vi "Create image name.vi"(8 "error in (no error)":errorcluster, 9 "Suffix":string, 10 "Channel":u8, 11 "Simulated_CCD_Camera in":refnum<class "Simulated_CCD_Camera.lvclass">) -> (0 "error out":errorcluster, 3 "Simulated_CCD_Camera out":refnum<class "Simulated_CCD_Camera.lvclass">)   [LabVIEW 2018, in "Simulated_CCD_Camera.lvclass"]
doc: "Create the image name\n\nThis name is composed by the following parts. First, there are the year, month, and day of the beginning of the night in the format YYYYMMDD. Second, there is the string s4cx, where x is the number of the channel. Then, there is the image index in the format 000000. This index is incremented after each acquisition. Finally, there is the suffix provided by the user. Following, there is an example of the image name\n\n20230101_s4c1_000001_zero.fits"
uses:
  Simulated_CCD_Camera.lvclass
  Simulated_CCD_Camera.lvclass/Simulated_CCD_Camera.ctl
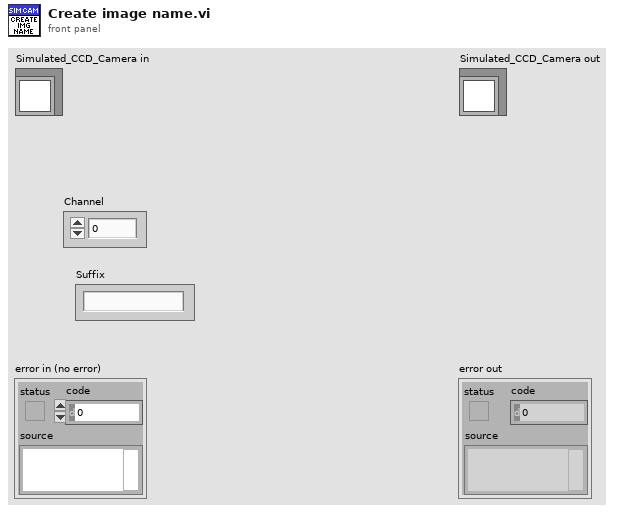
[diagram p1: front panel]
types:
  T1 = typedef "LVDateTimeRec.ctl" = cluster{"fractional second":dbl, "second":i32, "minute":i32, "hour":i32, "day of month":i32, "month":i32, "year":i32, "day of week":i32, "day of year":i32, "DST":i32}
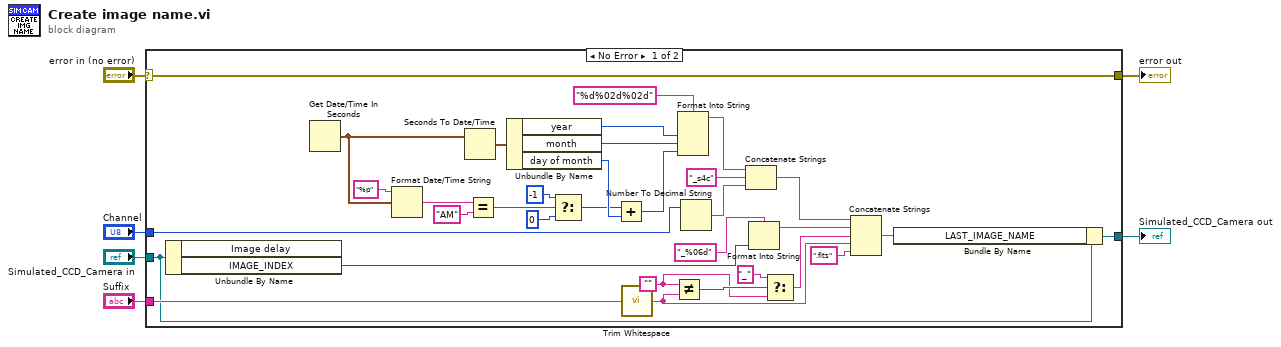
[diagram p0: block diagram]
diagram:
  n1 = case shown="No Error" "error in (no error)" {
    selector: "error in (no error)" -> [w11 w41]
    tunnel: [w11 w41] -> w5
    tunnel: [w29 w40] -> w3
    tunnel: "Simulated_CCD_Camera in" -> [w30 w40]
    tunnel: "Suffix" -> [w32 _]
    tunnel: "Channel" -> [w31 _]
    frame No Error {
      w26 = ""
      n2 = Unbundle By Name(w30) -> ("IMAGE_INDEX"=w22:u32)  [unwired: 1 out]
      n3 = Get Date/Time In Seconds() -> (seconds since 1Jan1904=w12:timestamp)
      n4 = Format Date/Time String(time format string (%c)="%p", seconds (now)=w12) -> (date/time string=w14:string)  [unwired: 1 in]
      n5 = Seconds To Date/Time(time stamp (now)=w12) -> (date time rec=w25:T1)  [unwired: 1 in]
      n6 = Equal?(x=w14, y="AM") -> (x = y?=w15:bool)
      n7 = Unbundle By Name(w25) -> ("year"=w24:i32, "month"=w23:i32, "day of month"=w19:i32)
      n8 = Select(t=-1, s=w15, f=0) -> (s? t:f=w18:i32)
      n9 = Add(x=w18, y=w19) -> (x+y=w17:i32)
      n10 = call <vilib>:"Trim Whitespace.vi"("string"=w32) -> ("trimmed string"=w9:string)  [unwired: 1 in]
      n11 = Not Equal?(x=w26, y=w9) -> (x != y?=w36:bool)
      n12 = Format Into String(format string="%d%02d%02d", w24, w23, w17) -> (resulting string=w27:string)  [unwired: 2 in, 1 out]
      n13 = Number To Decimal String(number=w31) -> (decimal integer string=w38:string)  [unwired: 1 in]
      n14 = Concatenate Strings(w27, "_s4c" ("string"), w38) -> (w37:string)
      n15 = Format Into String(format string="_%06d", w22) -> (resulting string=w8:string)  [unwired: 2 in, 1 out]
      n16 = Select(t="_" ("string"), s=w36, f=w26) -> (s? t:f=w7:string)
      n17 = Concatenate Strings(w37, w8, w7, w9, ".fits" ("string")) -> (w10:string)
      n18 = Bundle By Name(cluster=w30, "LAST_IMAGE_NAME"=w10) -> (w29:refnum<class "Simulated_CCD_Camera.lvclass">)
    }
    frame Error {
    }
  }
  "error out" <- w5
  "Simulated_CCD_Camera out" <- w3
